vi "Init.vi"(5 "Token Type":string, 7 "Scope":string, 10 "Refresh Token":string, 11 "Access Token":string) -> (3 "Authorization":refnum<class "Authorization.lvclass">)   [LabVIEW 2020, in "OAuth2.lvlib" / "Authorization.lvclass"]
uses:
  Authorization.lvclass
  Authorization.lvclass/Authorization.ctl
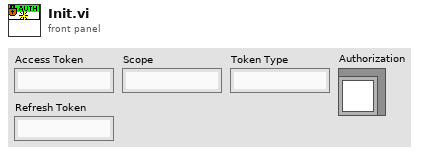
[diagram p1: front panel]
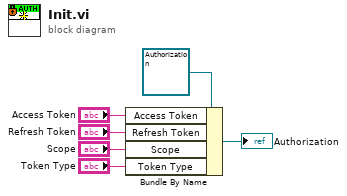
[diagram p0: block diagram]
diagram:
  n1 = Bundle By Name(cluster=refnum<class "Authorization.lvclass"> refnum ("OAuth2:Authorization"), "Access Token"="Access Token", "Refresh Token"="Refresh Token", "Scope"="Scope", "Token Type"="Token Type") -> (→"Authorization":refnum<class "Authorization.lvclass">)
